vi "Configure Synchronize Source.vi"(8 "error in (no error)":errorcluster, 9 "Synchronize Source (1: I1)":i32(ring)=1 items=["U1", "I1", "U2", "I2", "U3", "I3", "U4", "I4", "U5", "I5", "U6", "I6", "External Clock", "None"], 10 "Element/Wiring Unit (0: All)":i32(ring) items=["All", "1", "2", "3", "4", "5", "6", "Sigma A", "Sigma B", "Sigma C"], 11 "VISA resource name":refnum<visa-resource-name>) -> (0 "error out":errorcluster, 3 "VISA resource name out":refnum<visa-resource-name>)   [LabVIEW 2021, in "Yokogawa WT1800 Series.lvlib"]
doc: "Configures the synchronize source features."
uses:
  <instrlib>/Yokogawa WT1800 Series/Yokogawa WT1800 Series.lvlib
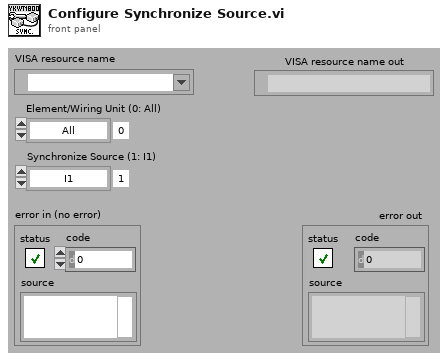
[diagram p1: front panel]
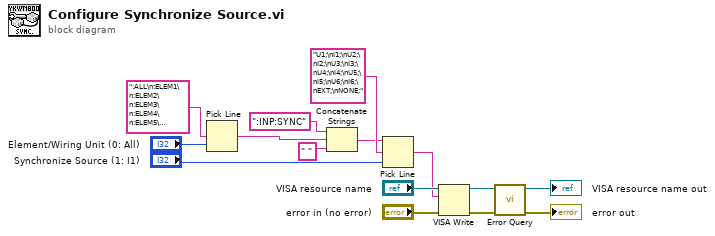
[diagram p0: block diagram]
diagram:
  n1 = Pick Line ("ライン選択")(multi-line string=":ALL\n:ELEM1\n:ELEM2\n:ELEM3\n:ELEM4\n:ELEM5\n:ELEM6\n:SIGMA\n:SIGMB\n:SIGMC" ("複数行文字列"), line index="Element/Wiring Unit (0: All)") -> (output string=w7:string)  [unwired: 1 in]
  n2 = Concatenate Strings(":INP:SYNC", w7, " " ("文字列")) -> (w4:string)
  n3 = Pick Line ("ライン選択")(string ("")=w4, multi-line string="U1;\nI1;\nU2;\nI2;\nU3;\nI3;\nU4;\nI4;\nU5;\nI5;\nU6;\nI6;\nEXT;\nNONE;" ("複数行文字列"), line index="Synchronize Source (1: I1)") -> (output string=w1:string)
  n4 = VISA Write ("VISA書き込み")(VISA resource name="VISA resource name", write buffer=w1, error in (no error)="error in (no error)") -> (VISA resource name out=w15:refnum<visa-resource-name>, error out=w14:errorcluster)  [unwired: 1 out]
  n5 = call <instrlib>:"Error Query.vi"("error in (no error)"=w14, "VISA resource name"=w15) -> ("error out"=→"error out":errorcluster, "VISA resource name out"=→"VISA resource name out":refnum<visa-resource-name>)  [unwired: 6 in, 2 out]
